vi "Set Pin Status.vi"(0 "UI Actor in":refnum<class "UI Actor.lvclass">, 5 "Puerto":string(combo), 7 "Pin":string(combo), 9 "Valor":string(combo), 11 "error in (no error)":errorcluster) -> (4 "UI Actor out":refnum<class "UI Actor.lvclass">, 15 "error out":errorcluster)   [LabVIEW 2020, in "UI Actor.lvlib" / "UI Actor.lvclass"]
uses:
  UI Actor.lvclass
  UI Actor.lvclass/UI Actor.ctl
  Abstract/Serial Device/Serial Device.lvclass
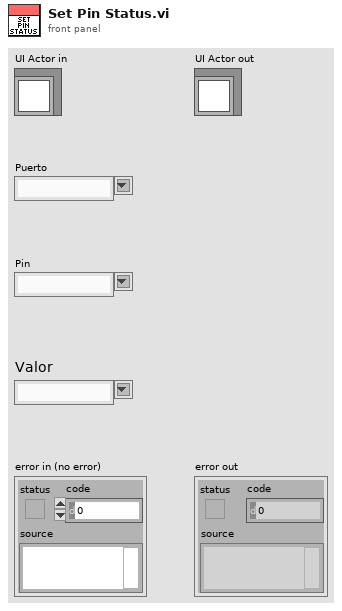
[diagram p1: front panel]
types:
  T1 = typedef "Control 1.ctl" = string
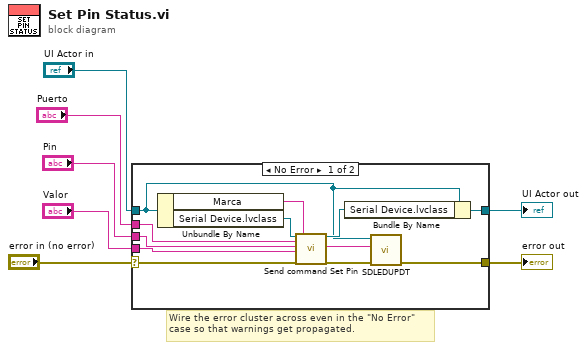
[diagram p0: block diagram]
diagram:
  # "Wire the error cluster across even in the \"No Error\"\ncase so that warnings get propagated."
  n1 = case shown="No Error" "error in (no error)" {
    selector: "error in (no error)" -> [w19 w21]
    tunnel: [w12 w21] -> w6
    tunnel: [w18 w20] -> w4
    tunnel: "UI Actor in" -> [w10 w20]
    tunnel: "Puerto" -> [w16 _]
    tunnel: "Pin" -> [w15 _]
    tunnel: "Valor" -> [w14 _]
    frame No Error {
      n2 = Unbundle By Name(w10) -> ("Marca"=w9:T1, "Serial Device.lvclass"=w8:refnum<class "Serial Device.lvclass">)
      n3 = call-dynamic "Send command Set Pin.vi"("Serial Device in"=w8, "Puerto"=w16, "Pin"=w15, "Valor"=w14, "error in (no error)"=w19, "Marca"=w9) -> ("Serial Device out"=w17:refnum<class "Serial Device.lvclass">, "Command"=w11:string, "error out"=w13:errorcluster)  [unwired: 10 in, 1 out]
      n4 = Bundle By Name(cluster=w10, "Serial Device.lvclass"=w17) -> (w18:refnum<class "UI Actor.lvclass">)
      n5 = call "SDLEDUPDT.vi"("error in (no error)"=w13, "Command"=w11, "UI Actor in"=w10) -> ("error out"=w12:errorcluster)  [unwired: 8 in]
    }
    frame Error {
    }
  }
  "error out" <- w6
  "UI Actor out" <- w4
